vi "McP789A-SimpleMove-v1.00.vi"(0 "New Counter Position":dbl=10000.0 min=0.0 max=26000.0 format="%.2f", 11 "error in (no error)":errorcluster, 13 "Grating factor":dbl=10.0 min=0.1 max=100.0 format="%.2f") -> (4 "Final CounterRdg":dbl=10000.0 min=0.0 max=26000.0 format="%.2f", 8 "Final Wavelenth(nm)":dbl=1000.0 format="%.2f", 10 "Final Stepper Position":i32=-1000000, 15 "error out":errorcluster)   [LabVIEW 2021]
doc: "McP 789A-3 mover. Needs new counter position and velocity input, it reads current counter position from disk and save the final position back to disk."
uses:
  Globals and TypeDefs/Global Varibal Control.vi
panel:
  out "Current Couter Reading":dbl=-1125000.0 format="%.2f"
  out "Current Stepper Position":i32=-1125000
  out "Current stepPos":i32=-1125000
  out "New Wavelength(nm)":dbl=1000.0 min=0.0 max=100000.0 format="%.3f"
  out "DelayTime":dbl=10.0 format="%.3f"
  out "Current CounterRdg":dbl=9500.0 min=0.0 max=26000.0 format="%.3f"
  out "Current Wavelength(nm)":dbl=950.0 min=0.0 max=100000.0 format="%.3f"
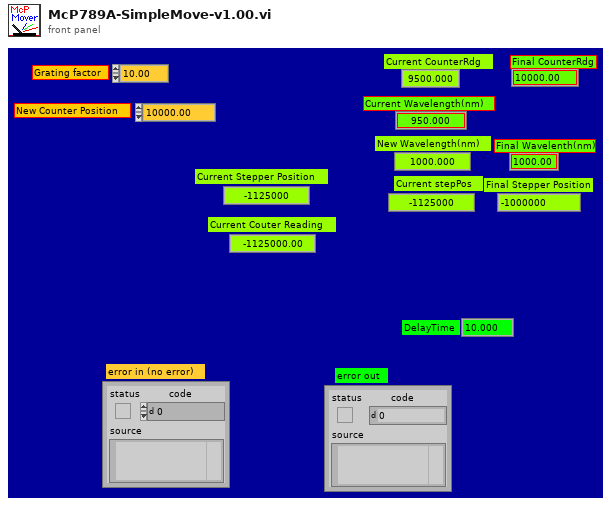
[diagram p1: front panel]
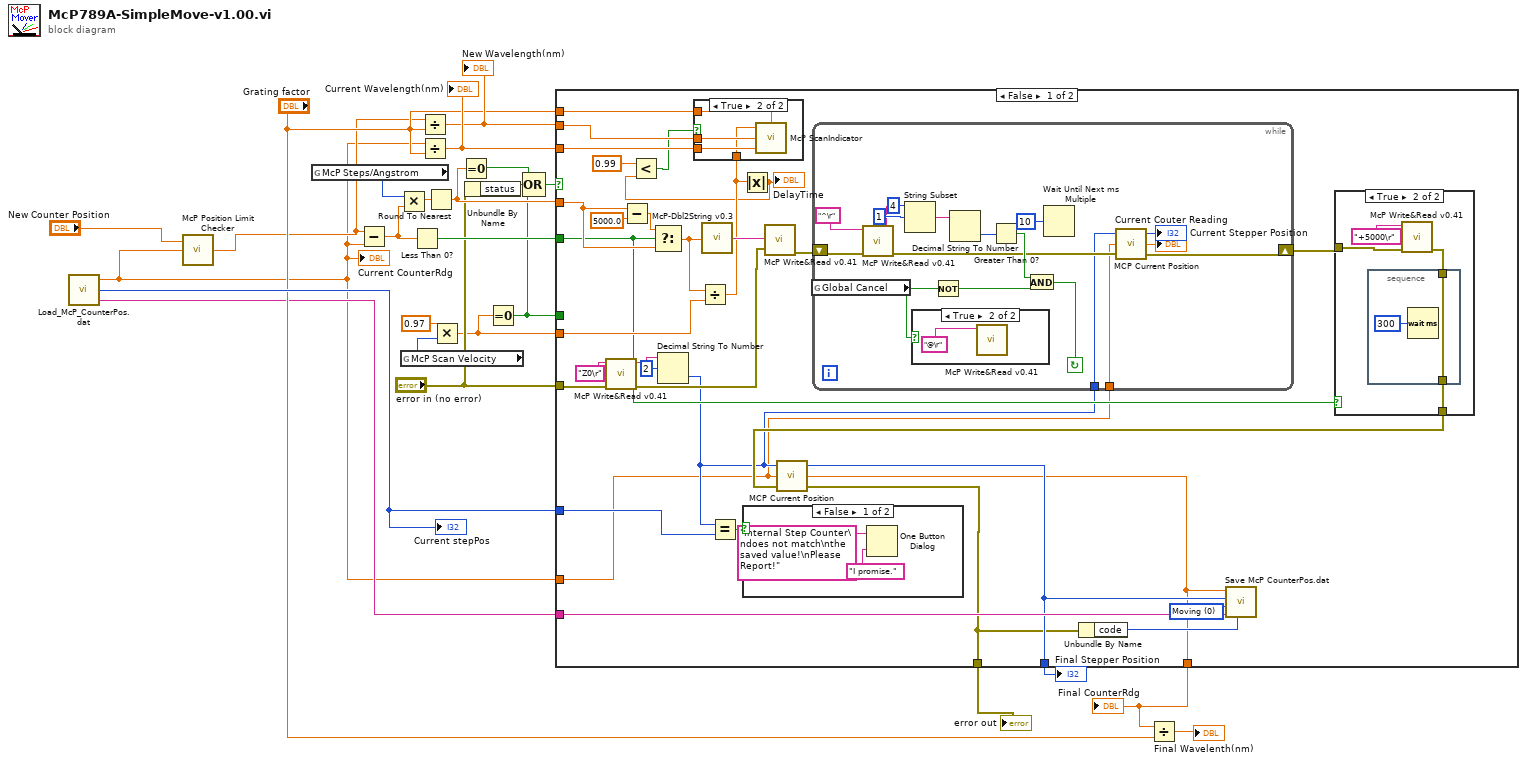
[diagram p0: block diagram]
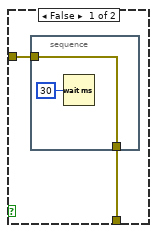
[diagram p5: hidden frame]
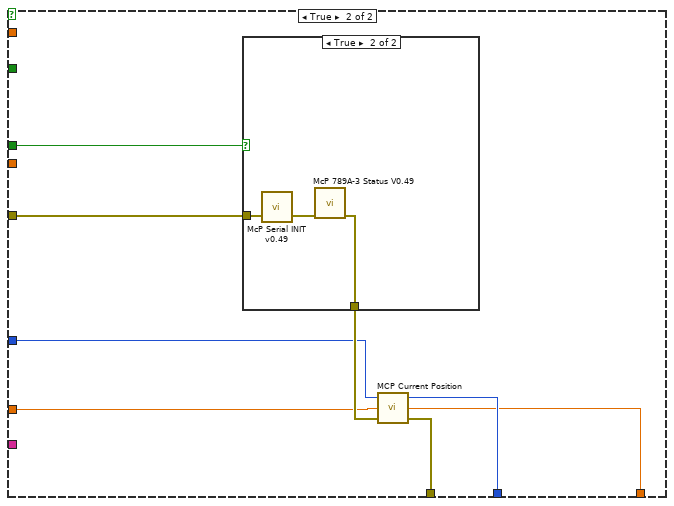
[diagram p6: hidden frame]
diagram:
  n1 = call "Load_McP_CounterPos.dat.vi"() -> ("Counter Position"=w1:dbl, "Stepper Position"=w22:i32, "Last Calibration Date"=w8:string)  [unwired: 1 in]
  "Current CounterRdg" <- w1
  "Current stepPos" <- w22
  n2 = call "McP Position Limit Checker.vi"("Old Counter Position"=w1, "New Counter Position"="New Counter Position") -> ("New Counter Position output"=w3:dbl)  [unwired: 1 in]
  n3 = global read "Global Varibal Control.vi" "McP Steps/Angstrom"() -> (w5:i32)
  n4 = Subtract(x=w3, y=w1) -> (x-y=w23:dbl)
  n5 = Multiply(x=w5, y=w23) -> (x*y=w18:dbl)
  n6 = global read "Global Varibal Control.vi" "McP Scan Velocity"() -> (w4:i32)
  n7 = Less Than 0?(x=w23) -> (x < 0?=w24:bool)
  n8 = Divide(x=w3, y="Grating factor") -> (x/y=w20:dbl)
  "New Wavelength(nm)" <- w20
  n9 = Divide(x=w1, y="Grating factor") -> (x/y=w21:dbl)
  "Current Wavelength(nm)" <- w21
  n10 = Round To Nearest(number=w18) -> (nearest integer value=w17:dbl)
  n11 = Multiply(x=0.97, y=w4) -> (x*y=w7:dbl)
  n12 = Equal To 0?(x=w17) -> (x = 0?=w13:bool)
  n13 = Unbundle By Name("error in (no error)") -> ("status"=w14:bool)
  n14 = Equal To 0?(x=w7) -> (x = 0?=w6:bool)
  n15 = Compound Arithmetic op=OR(w13, w14, w6) -> (w12:bool)
  n16 = case shown="False" w12 {
    tunnel: w24 -> [w51 _]
    tunnel: w17 -> [w56 _]
    tunnel: w7 -> [w52 _]
    tunnel: "Grating factor" -> [w40 _]
    tunnel: w20 -> [w38 _]
    tunnel: w21 -> [w39 _]
    tunnel: w22 -> [w45 w96]
    tunnel: w1 -> [w26 w97]
    tunnel: [w34 w94] -> w10
    tunnel: "error in (no error)" -> [w47 w99]
    tunnel: [w35 w95] -> w9
    tunnel: [w32 w93] -> w16
    tunnel: w8 -> [w42 _]
    tunnel: w6 -> [_ w100]
    frame False {
      w41 = u16 0 items=["Moving", "Calibration", "Key in", "Initialization"] ("Set Method")
      n17 = call "McP Write&Read v0.41.vi"("error in (no error)"=w47, "Write String"="Z0\r") -> ("error out"=w46:errorcluster, "Read String\nshows:"=w49:string)  [unwired: 2 in, 3 out]
      n18 = Subtract(x=w56, y=5000.0) -> (x-y=w55:dbl)
      n19 = Select(t=w55, s=w51, f=w56) -> (s? t:f=w53:dbl)
      n20 = Decimal String To Number(string=w49, offset=2) -> (number=w27:i32)  [unwired: 1 in, 1 out]
      n21 = Divide(x=w53, y=w52) -> (x/y=w29:dbl)
      n22 = call "McP-Dbl2String v0.3.vi"("McP Input Number"=w53) -> ("Controller String"=w54:string)
      n23 = Equal?(x=w27, y=w45) -> (x = y?=w44:bool)
      n24 = Absolute Value(x=w29) -> (abs(x)=w28:dbl)
      "DelayTime" <- w28
      n25 = Less?(x=0.99, y=w28) -> (x < y?=w30:bool)
      n26 = case shown="True" w30 {
        tunnel: w40 -> [_ w80]
        tunnel: w39 -> [_ w79]
        tunnel: w38 -> [_ w78]
        tunnel: w29 -> [_ w77]
        frame False {
        }
        frame True {
          n27 = call "McP ScanIndicator.vi"("Grating factor"=w80, "Current Wavelength"=w79, "New Wavelength"=w78, "MoveTime(ms)"=w77) -> ()  [unwired: 1 in]
        }
      }
      n28 = case shown="False" w44 {
        frame False {
          n29 = One Button Dialog(message="Internal Step Counter\ndoes not match\nthe saved value!\nPlease Report!", button name ("OK")="I promise.") -> ()  [unwired: 1 out]
        }
        frame True {
        }
      }
      n30 = call "McP Write&Read v0.41.vi"("error in (no error)"=w46, "Write String"=w54) -> ("error out"=w37:errorcluster)  [unwired: 2 in, 4 out]
      n31 = while {
        tunnel: w26 -> [w60]
        tunnel: w27 -> [w61]
        shift-left: w37 -> [w75]
        shift-right: [w62] -> w36
        stop <- w67 continue-if-true
        n32 = global read "Global Varibal Control.vi" "Global Cancel"() -> (w64:bool)
        n33 = call "McP Write&Read v0.41.vi"("error in (no error)"=w75, "Write String"="^\r") -> ("error out"=w63:errorcluster, "Read String\nshows:"=w71:string)  [unwired: 2 in, 3 out]
        n34 = String Subset(string=w71, offset (0)=1, length (rest)=4) -> (substring=w70:string)
        n35 = case shown="True" w64 {
          frame False {
          }
          frame True {
            n36 = call "McP Write&Read v0.41.vi"("Write String"="@\r") -> ()  [unwired: 3 in, 5 out]
          }
        }
        n37 = Not(x=w64) -> (.not. x?=w65:bool)
        n38 = Decimal String To Number(string=w70) -> (number=w68:i32)  [unwired: 2 in, 1 out]
        n39 = Greater Than 0?(x=w68) -> (x > 0?=w66:bool)
        n40 = And(x=w66, y=w65) -> (x .and. y?=w67:bool)
        n41 = Wait Until Next ms Multiple(millisecond multiple=u32 10) -> ()  [unwired: 1 out]
        n42 = call "MCP Current Position.vi"("error in (no error)"=w63, "Initial Couter Reading"=w60, "Initial Stepper Position"=w61) -> ("error out"=w62:errorcluster, "Current Couter Reading"=→"Current Couter Reading":dbl, "Current Stepper Position"=→"Current Stepper Position":i32)
      }
      n43 = case shown="True" w51 {
        tunnel: w36 -> [w84 w89]
        tunnel: [w83 w87] -> w33
        frame False {
          n44 = stacked-sequence {
            tunnel: [w85] -> w83
            tunnel: w84 -> [w85]
            frame #0 {
              n45 = Wait (ms)(milliseconds to wait=u32 30) -> ()  [unwired: 1 out]
            }
          }
        }
        frame True {
          n46 = call "McP Write&Read v0.41.vi"("error in (no error)"=w89, "Write String"="+5000\r") -> ("error out"=w88:errorcluster)  [unwired: 2 in, 4 out]
          n47 = stacked-sequence {
            tunnel: w88 -> [w91]
            tunnel: [w91] -> w87
            frame #0 {
              n48 = Wait (ms)(milliseconds to wait=u32 300) -> ()  [unwired: 1 out]
            }
          }
        }
      }
      n49 = call "MCP Current Position.vi"("error in (no error)"=w33, "Initial Couter Reading"=w26, "Initial Stepper Position"=w27) -> ("error out"=w32:errorcluster, "Current Couter Reading"=w34:dbl, "Current Stepper Position"=w35:i32)
      n50 = Unbundle By Name(w32) -> ("code"=w43:i32)
      n51 = call "Save McP CounterPos.dat.vi"("Error Code (0: No Error)"=w43, "Last Calibration Date"=w42, "Set Method"=w41, "McP Stepper Position"=w35, "McP Counter Position"=w34) -> ()  [unwired: 1 in, 1 out]
    }
    frame True {
      n52 = case shown="True" w100 {
        tunnel: w99 -> [w101 w103]
        tunnel: [w101 w102] -> w98
        frame False {
        }
        frame True {
          n53 = call "McP Serial INIT v0.49.vi"("error in (no error)"=w103) -> ("Error out"=w104:errorcluster)  [unwired: 1 in, 1 out]
          n54 = call "McP 789A-3 Status V0.49.vi"("error in (no error)"=w104) -> ("error out"=w102:errorcluster)  [unwired: 7 in, 3 out]
        }
      }
      n55 = call "MCP Current Position.vi"("error in (no error)"=w98, "Initial Couter Reading"=w97, "Initial Stepper Position"=w96) -> ("error out"=w93:errorcluster, "Current Couter Reading"=w94:dbl, "Current Stepper Position"=w95:i32)
    }
  }
  "Final CounterRdg" <- w10
  "Final Stepper Position" <- w9
  "error out" <- w16
  n56 = Divide(x=w10, y="Grating factor") -> (x/y=→"Final Wavelenth(nm)":dbl)
